vi "FilterOrphanFolder.vi"(11 "TreeCluster":T1(array[cluster])) -> (3 "TreeCluster 2":T1(array[cluster]))   [LabVIEW 2013, in "FindName Task_Manager.lvlib"]
uses:
  FindName Task_Manager.lvlib
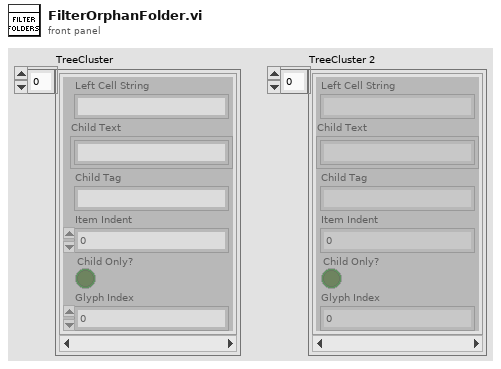
[diagram p1: front panel]
types:
  T1 = cluster{"Left Cell String":string, "Child Text":string[], "Child Tag":string, "Item Indent":i32, "Child Only?":bool, "Glyph Index":i32}[]
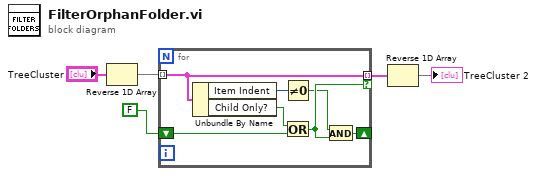
[diagram p0: block diagram]
diagram:
  n1 = Reverse 1D Array(array="TreeCluster") -> (reversed array=w4:T1)
  n2 = for {
    tunnel: w4 -> [w12] mode=indexing
    tunnel: [w12] -> w2 mode=indexing if=w8
    shift-right: [w6] -> _
    shift-left: FALSE ("Child Only?") -> [w9]
    n3 = Unbundle By Name(w12) -> ("Item Indent"=w11:i32, "Child Only?"=w10:bool)
    n4 = Not Equal To 0?(x=w11) -> (x != 0?=w7:bool)
    n5 = Or(x=w10, y=w9) -> (x .or. y?=w8:bool)
    n6 = And(x=w7, y=w8) -> (x .and. y?=w6:bool)
  }
  n7 = Reverse 1D Array(array=w2) -> (reversed array=→"TreeCluster 2":T1)
